vi "BMark_GetDisplayableItemName.vi"(9 "file or folder":string, 10 "parent folder":path) -> (2 "display name":string)   [LabVIEW 2016]
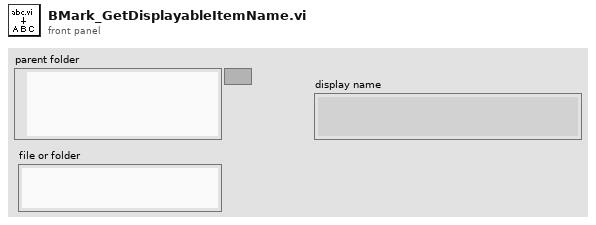
[diagram p1: front panel]
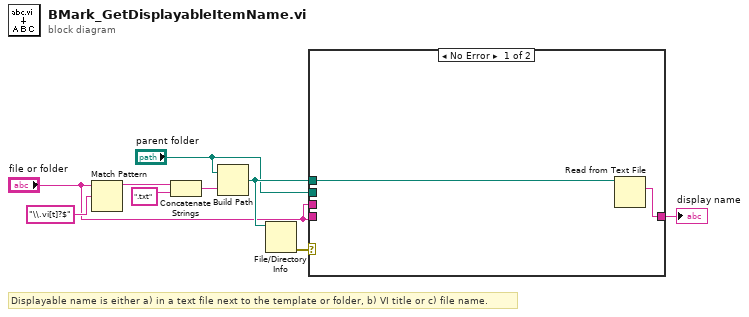
[diagram p0: block diagram]
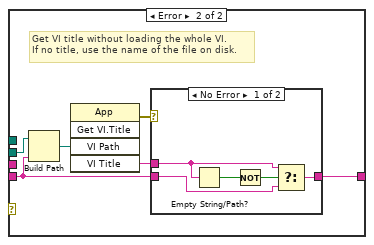
[diagram p2: hidden frame]
diagram:
  # "Displayable name is either a) in a text file next to the template or folder, b) VI title or c) file name."
  n1 = Match Pattern(string="file or folder", regular expression="\\.vi[t]?$") -> (before substring=w5:string)  [unwired: 1 in, 3 out]
  n2 = Concatenate Strings(w5, ".txt" ("string")) -> (w7:string)
  n3 = Build Path(base path="parent folder", name or relative path=w7) -> (appended path=w8:path)
  n4 = File/Directory Info(path=w8) -> (error out=w9:errorcluster)  [unwired: 1 in, 6 out]
  n5 = case shown="No Error" w9 {
    tunnel: w8 -> [w11 _]
    tunnel: "file or folder" -> [_ _]
    tunnel: "parent folder" -> [_ w17]
    tunnel: "file or folder" -> [_ w12]
    tunnel: [w10 w13] -> w1
    frame No Error {
      n6 = Read from Text File(file (use dialog)=w11) -> (text=w10:string)  [unwired: 3 in, 3 out]
    }
    frame Error {
      # "Get VI title without loading the whole VI.\nIf no title, use the name of the file on disk."
      n7 = Build Path(base path=w17, name or relative path=w12) -> (appended path=w16:path)
      n8 = invoke class="App" method="Get VI.Title"("VI Path"=w16) -> (error out=w15:errorcluster, "VI Title"=w14:string)  [unwired: 4 in, 3 out]
      n9 = case shown="No Error" w15 {
        tunnel: [w18 w23] -> w13
        tunnel: w14 -> [w20 _]
        tunnel: w12 -> [w19 w23]
        frame No Error {
          n10 = Empty String/Path?(string/path=w20) -> (empty?=w22:bool)
          n11 = Not(x=w22) -> (.not. x?=w21:bool)
          n12 = Select(t=w20, s=w21, f=w19) -> (s? t:f=w18:string)
        }
        frame Error {
        }
      }
    }
  }
  "display name" <- w1
